vi "update_track_snippet.vi"(8 "Input Track Snippet":T1={"Track Centroid Positions (Camera Pixel)"=[], "Within Track Index"=0, "Camera Buffer Indecies"=[], "Area (Camera Pixels)"=0, "Speed (mm/s)"=0.0, "Direction (radians)"=0.0, "Centerline Positions (Camera Pixel)"=[], "Ellipse Ratio"=0.0, "Termination Reason"=enum."StillActive", "Track Index"=0, "Bounding Rect Left"=0, "Bounding Rect Top"=0, "Bounding Rect Right"=0, "Bounding Rect Bottom"=0, "Mature Camera Buffer"=-1, "Start Camera Buffer Index"=0, "Reverse Started Camera Buffer"=-1}, 9 "Current Camera Buffer Number":i32, 11 "Particle Analysis Output":dbl[](array[numeric])) -> (0 "Output Track Snippet":T1={"Track Centroid Positions (Camera Pixel)"=[], "Within Track Index"=0, "Camera Buffer Indecies"=[], "Area (Camera Pixels)"=0, "Speed (mm/s)"=0.0, "Direction (radians)"=0.0, "Centerline Positions (Camera Pixel)"=[], "Ellipse Ratio"=0.0, "Termination Reason"=enum."StillActive", "Track Index"=0, "Bounding Rect Left"=0, "Bounding Rect Top"=0, "Bounding Rect Right"=0, "Bounding Rect Bottom"=0, "Mature Camera Buffer"=-1, "Start Camera Buffer Index"=0, "Reverse Started Camera Buffer"=-1})   [LabVIEW 2019]
uses:
  WormTrackSnippetCluster.ctl
  TrackTerminationReasonEnum.ctl
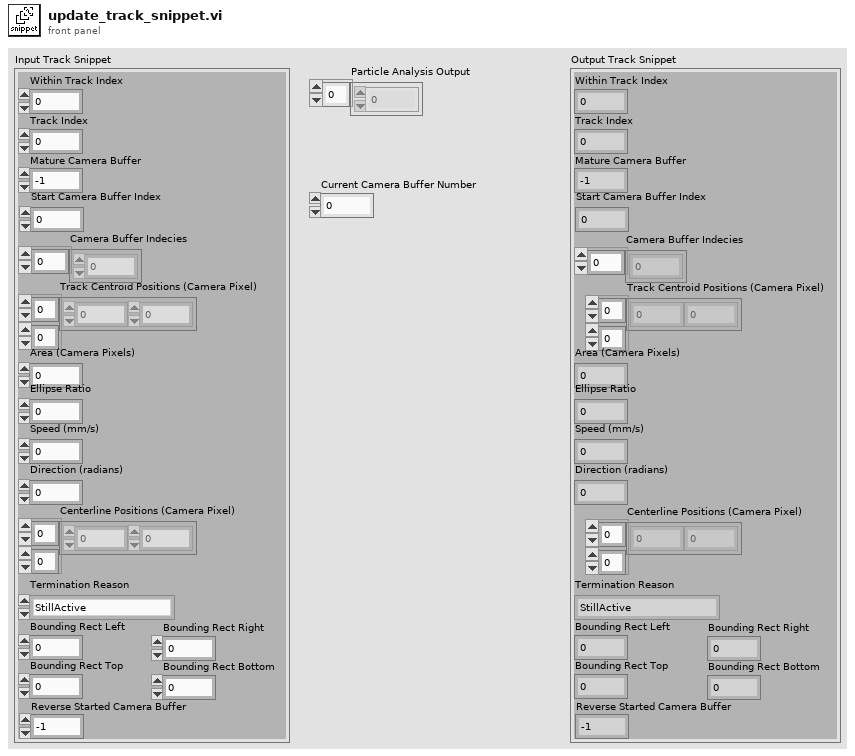
[diagram p1: front panel]
types:
  T1 = typedef "WormTrackSnippetCluster.ctl" = cluster{"Track Centroid Positions (Camera Pixel)":sgl[][], "Within Track Index":i32, "Camera Buffer Indecies":i32[], "Area (Camera Pixels)":i32, "Speed (mm/s)":sgl, "Direction (radians)":sgl, "Centerline Positions (Camera Pixel)":sgl[][], "Ellipse Ratio":sgl, "Termination Reason":T2, "Track Index":i32, "Bounding Rect Left":i32, "Bounding Rect Top":i32, "Bounding Rect Right":i32, "Bounding Rect Bottom":i32, "Mature Camera Buffer":i32, "Start Camera Buffer Index":i32, "Reverse Started Camera Buffer":i32}
  T2 = typedef "TrackTerminationReasonEnum.ctl" = enum16{"StillActive", "MaxDisplacement", "NoBlobsLeft", "AreaIncrease", "AreaDecrease", "ExperimentEnded"}
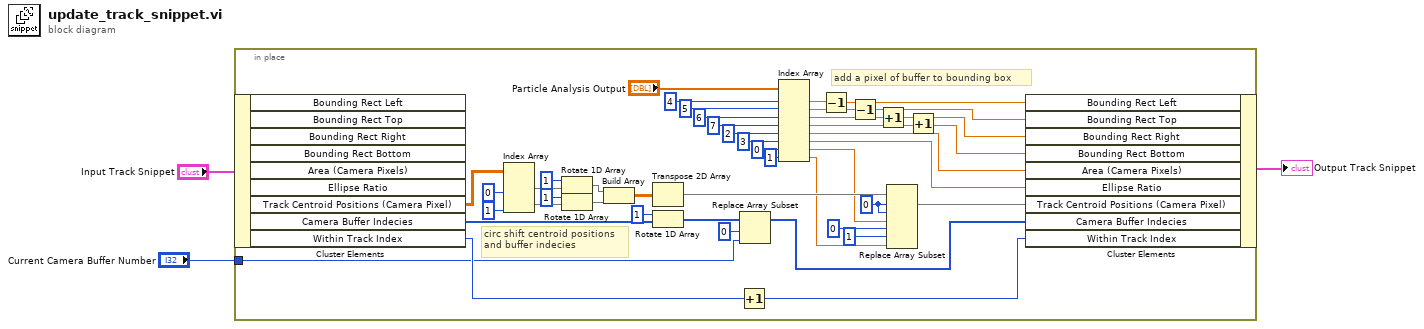
[diagram p0: block diagram]
diagram:
  n1 = in-place {
    in-place-border: "Current Camera Buffer Number" -> [w4]
    w12 = 0 ("index (row)")
    # "circ shift centroid positions\nand buffer indecies"
    # "add a pixel of buffer to bounding box"
    n2 = in-place-cluster #1("Input Track Snippet") -> ("Track Centroid Positions (Camera Pixel)"=w25:sgl[][], "Camera Buffer Indecies"=w27:i32[], "Within Track Index"=w28:i32)  [unwired: 6 out]
    n3 = Index Array(array=w25, index (col) #1=0 ("disabled index (col)"), index (col) #2=1 ("index (col)")) -> (element #1=w21:sgl[], element #2=w19:sgl[])  [unwired: 2 in]
    n4 = Rotate 1D Array(1:w21, 2:1 ("n")) -> (0:w18:sgl[])
    n5 = Rotate 1D Array(1:w19, 2:1 ("n")) -> (0:w17:sgl[])
    n6 = Build Array(w18, w17) -> (w16:sgl[][])
    n7 = Transpose 2D Array(2D array=w16) -> (transposed array=w15:sgl[][])
    n8 = Rotate 1D Array(1:w27, 2:1 ("n")) -> (0:w7:i32[])
    n9 = Increment(x=w28) -> (x+1=w8:i32)
    n10 = Replace Array Subset(array=w7, new element=w4, index=0) -> (w5:i32[])
    n11 = Index Array(array="Particle Analysis Output", index #1=4 ("index"), index #2=5 ("index"), index #3=6 ("index"), index #4=7 ("index"), index #5=2 ("index"), index #6=3 ("index"), index #7=0 ("index"), index #8=1 ("index")) -> (element #1=w38:dbl, element #2=w37:dbl, element #3=w34:dbl, element #4=w32:dbl, element #5=w30:dbl, element #6=w29:dbl, element #7=w10:dbl, element #8=w9:dbl)
    n12 = Decrement(x=w38) -> (x-1=w36:dbl)
    n13 = Decrement(x=w37) -> (x-1=w35:dbl)
    n14 = Increment(x=w34) -> (x+1=w33:dbl)
    n15 = Replace Array Subset(array=w15, new element #1=w10, index (row) #1=w12, index (col) #1=w12, new element #2=w9, index (row) #2=0 ("index (row)"), index (col) #2=1 ("disabled index (col)")) -> (w14:sgl[][])
    n16 = Increment(x=w32) -> (x+1=w31:dbl)
    n17 = in-place-cluster #1("Bounding Rect Left"=w36, "Bounding Rect Top"=w35, "Bounding Rect Right"=w33, "Bounding Rect Bottom"=w31, "Area (Camera Pixels)"=w30, "Ellipse Ratio"=w29, "Track Centroid Positions (Camera Pixel)"=w14, "Camera Buffer Indecies"=w5, "Within Track Index"=w8) -> (→"Output Track Snippet":T1)
  }
